vi "GeoData.vi"() -> ()   [LabVIEW 2017] (continued)
\tPembine\tWI\tMarinette County\tH1\n54151\t55075\tNiagara\tWI\tMarinette County\tH1\n54153\t55075\tOconto\tWI\tMarinette County\tH1\n54112\t55075\tColeman\tWI\tMarinette County\tH1\n54125\t55075\tGoodman\tWI\tMarinette County\tH1\n54119\t55075\tDunbar\tWI\tMarinette County\tH1\n54143\t55075\tMarinette\tWI\tMarinette County\tH1\n54139\t55075\tLena\tWI\tMarinette County\tH1\n54120\t55075\tFence\tWI\tMarinette County\tH1\n54159\t55075\tPorterfield\tWI\tMarinette County\tH1\n54103\t55075\tArmstrong creek\tWI\tMarinette County\tH1\n54114\t55075\tCrivitz\tWI\tMarinette County\tH1\n54102\t55075\tAmberg\tWI\tMarinette County\tH1\n54177\t55075\tWausaukee\tWI\tMarinette County\tH1\n54104\t55075\tAthelstane\tWI\tMarinette County\tH1\n53949\t55077\tMontello\tWI\tMarquette County\tH1\n53953\t55077\tPackwaukee\tWI\tMarquette County\tH1\n53954\t55077\tPardeeville\tWI\tMarquette County\tH1\n53930\t55077\tEndeavor\tWI\tMarquette County\tH1\n54930\t55077\tColoma\tWI\tMarquette County\tH1\n53946\t55077\tMarkesan\tWI\tMarquette County\tH1\n53920\t55077\tBriggsville\tWI\tMarquette County\tH1\n53901\t55077\tPortage\tWI\tMarquette County\tH1\n53952\t55077\tOxford\tWI\tMarquette County\tH1\n53926\t55077\tDalton\tWI\tMarquette County\tH1\n54960\t55077\tNeshkoro\tWI\tMarquette County\tH1\n54982\t55077\tWautoma\tWI\tMarquette County\tH1\n54968\t55077\tPrinceton\tWI\tMarquette County\tH1\n53964\t55077\tWestfield\tWI\tMarquette County\tH1\n54135\t55078\tKeshena\tWI\tMenominee County\tH1\n54166\t55078\tShawano\tWI\tMenominee County\tH1\n54174\t55078\tSuring\tWI\tMenominee County\tH1\n54124\t55078\tGillett\tWI\tMenominee County\tH1\n54150\t55078\tNeopit\tWI\tMenominee County\tH1\n53217\t55079\tMilwaukee\tWI\tMilwaukee County\tH1\n53220\t55079\tMilwaukee\tWI\tMilwaukee County\tH1\n53235\t55079\tSaint francis\tWI\tMilwaukee County\tH1\n53226\t55079\tMilwaukee\tWI\tMilwaukee County\tH1\n53221\t55079\tMilwaukee\tWI\tMilwaukee County\tH1\n53154\t55079\tOak creek\tWI\tMilwaukee County\tH1\n53204\t55079\tMilwaukee\tWI\tMilwaukee County\tH1\n53132\t55079\tFranklin\tWI\tMilwaukee County\tH1\n53219\t55079\tMilwaukee\tWI\tMilwaukee County\tH1\n53203\t55079\tMilwaukee\tWI\tMilwaukee County\tH1\n53207\t55079\tMilwaukee\tWI\tMilwaukee County\tH1\n53212\t55079\tMilwaukee\tWI\tMilwaukee County\tH1\n53007\t55079\tButler\tWI\tMilwaukee County\tH1\n53233\t55079\tMilwaukee\tWI\tMilwaukee County\tH1\n53202\t55079\tMilwaukee\tWI\tMilwaukee County\tH1\n53206\t55079\tMilwaukee\tWI\tMilwaukee County\tH1\n53172\t55079\tSouth milwaukee\tWI\tMilwaukee County\tH1\n53210\t55079\tMilwaukee\tWI\tMilwaukee County\tH1\n53215\t55079\tMilwaukee\tWI\tMilwaukee County\tH1\n53263\t55079\tMilwaukee\tWI\tMilwaukee County\tH1\n53129\t55079\tGreendale\tWI\tMilwaukee County\tH1\n53228\t55079\tMilwaukee\tWI\tMilwaukee County\tH1\n53216\t55079\tMilwaukee\tWI\tMilwaukee County\tH1\n53234\t55079\tMilwaukee\tWI\tMilwaukee County\tH1\n53237\t55079\tMilwaukee\tWI\tMilwaukee County\tH1\n53213\t55079\tMilwaukee\tWI\tMilwaukee County\tH1\n53201\t55079\tMilwaukee\tWI\tMilwaukee County\tH1\n53293\t55079\tMilwaukee\tWI\tMilwaukee County\tH1\n53274\t55079\tMilwaukee\tWI\tMilwaukee County\tH1\n53110\t55079\tCudahy\tWI\tMilwaukee County\tH1\n53130\t55079\tHales corners\tWI\tMilwaukee County\tH1\n53126\t55079\tFranksville\tWI\tMilwaukee County\tH1\n53225\t55079\tMilwaukee\tWI\tMilwaukee County\tH1\n53224\t55079\tMilwaukee\tWI\tMilwaukee County\tH1\n53223\t55079\tMilwaukee\tWI\tMilwaukee County\tH1\n53211\t55079\tMilwaukee\tWI\tMilwaukee County\tH1\n53214\t55079\tMilwaukee\tWI\tMilwaukee County\tH1\n53295\t55079\tMilwaukee\tWI\tMilwaukee County\tH1\n53278\t55079\tMilwaukee\tWI\tMilwaukee County\tH1\n53222\t55079\tMilwaukee\tWI\tMilwaukee County\tH1\n53209\t55079\tMilwaukee\tWI\tMilwaukee County\tH1\n53208\t55079\tMilwaukee\tWI\tMilwaukee County\tH1\n53218\t55079\tMilwaukee\tWI\tMilwaukee County\tH1\n53227\t55079\tMilwaukee\tWI\tMilwaukee County\tH1\n53205\t55079\tMilwaukee\tWI\tMilwaukee County\tH1\n53259\t55079\tMilwaukee\tWI\tMilwaukee County\tH1\n54618\t55081\tCamp douglas\tWI\tMonroe County\tH1\n54666\t55081\tWarrens\tWI\tMonroe County\tH1\n54648\t55081\tNorwalk\tWI\tMonroe County\tH1\n54651\t55081\tOntario\tWI\tMonroe County\tH1\n53929\t55081\tElroy\tWI\tMonroe County\tH1\n54670\t55081\tWilton\tWI\tMonroe County\tH1\n54660\t55081\tTomah\tWI\tMonroe County\tH1\n54656\t55081\tSparta\tWI\tMonroe County\tH1\n54653\t55081\tRockland\tWI\tMonroe County\tH1\n54649\t55081\tOakdale\tWI\tMonroe County\tH1\n54619\t55081\tCashton\tWI\tMonroe County\tH1\n54615\t55081\tBlack river falls\tWI\tMonroe County\tH1\n54662\t55081\tTunnel city\tWI\tMonroe County\tH1\n54614\t55081\tBangor\tWI\tMonroe County\tH1\n54638\t55081\tKendall\tWI\tMonroe County\tH1\n54620\t55081\tCataract\tWI\tMonroe County\tH1\n54157\t55083\tPeshtigo\tWI\tOconto County\tH1\n54111\t55083\tCecil\tWI\tOconto County\tH1\n54161\t55083\tPound\tWI\tOconto County\tH1\n54491\t55083\tWhite lake\tWI\tOconto County\tH1\n54153\t55083\tOconto\tWI\tOconto County\tH1\n54112\t55083\tColeman\tWI\tOconto County\tH1\n54137\t55083\tKrakow\tWI\tOconto County\tH1\n54174\t55083\tSuring\tWI\tOconto County\tH1\n54171\t55083\tSobieski\tWI\tOconto County\tH1\n54141\t55083\tLittle suamico\tWI\tOconto County\tH1\n54124\t55083\tGillett\tWI\tOconto County\tH1\n54149\t55083\tMountain\tWI\tOconto County\tH1\n54154\t55083\tOconto falls\tWI\tOconto County\tH1\n54139\t55083\tLena\tWI\tOconto County\tH1\n54175\t55083\tTownsend\tWI\tOconto County\tH1\n54101\t55083\tAbrams\tWI\tOconto County\tH1\n54114\t55083\tCrivitz\tWI\tOconto County\tH1\n54162\t55083\tPulaski\tWI\tOconto County\tH1\n54138\t55083\tLakewood\tWI\tOconto County\tH1\n54104\t55083\tAthelstane\tWI\tOconto County\tH1\n54538\t55085\tLac du flambeau\tWI\tOneida County\tH1\n54529\t55085\tHarshaw\tWI\tOneida County\tH1\n54564\t55085\tTripoli\tWI\tOneida County\tH1\n54543\t55085\tMc naughton\tWI\tOneida County\tH1\n54539\t55085\tLake tomahawk\tWI\tOneida County\tH1\n54558\t55085\tSaint germain\tWI\tOneida County\tH1\n54521\t55085\tEagle river\tWI\tOneida County\tH1\n54501\t55085\tRhinelander\tWI\tOneida County\tH1\n54428\t55085\tElcho\tWI\tOneida County\tH1\n54562\t55085\tThree lakes\tWI\tOneida County\tH1\n54548\t55085\tMinocqua\tWI\tOneida County\tH1\n54531\t55085\tHazelhurst\tWI\tOneida County\tH1\n54463\t55085\tPelican lake\tWI\tOneida County\tH1\n54568\t55085\tWoodruff\tWI\tOneida County\tH1\n54435\t55085\tGleason\tWI\tOneida County\tH1\n54487\t55085\tTomahawk\tWI\tOneida County\tH1\n54520\t55085\tCrandon\tWI\tOneida County\tH1\n54914\t55087\tAppleton\tWI\tOutagamie County\tH1\n54942\t55087\tGreenville\tWI\tOutagamie County\tH1\n54130\t55087\tKaukauna\tWI\tOutagamie County\tH1\n54155\t55087\tOneida\tWI\tOutagamie County\tH1\n54152\t55087\tNichols\tWI\tOutagamie County\tH1\n54180\t55087\tWrightstown\tWI\tOutagamie County\tH1\n54922\t55087\tBear creek\tWI\tOutagamie County\tH1\n54961\t55087\tNew london\tWI\tOutagamie County\tH1\n54940\t55087\tFremont\tWI\tOutagamie County\tH1\n54106\t55087\tBlack creek\tWI\tOutagamie County\tH1\n54956\t55087\tNeenah\tWI\tOutagamie County\tH1\n54115\t55087\tDe pere\tWI\tOutagamie County\tH1\n54913\t55087\tAppleton\tWI\tOutagamie County\tH1\n54107\t55087\tBonduel\tWI\tOutagamie County\tH1\n54113\t55087\tCombined locks\tWI\tOutagamie County\tH1\n54313\t55087\tGreen bay\tWI\tOutagamie County\tH1\n54919\t55087\tAppleton\tWI\tOutagamie County\tH1\n54136\t55087\tKimberly\tWI\tOutagamie County\tH1\n54140\t55087\tLittle chute\tWI\tOutagamie County\tH1\n54165\t55087\tSeymour\tWI\tOutagamie County\tH1\n54911\t55087\tAppleton\tWI\tOutagamie County\tH1\n54915\t55087\tAppleton\tWI\tOutagamie County\tH1\n54931\t55087\tDale\tWI\tOutagamie County\tH1\n54170\t55087\tShiocton\tWI\tOutagamie County\tH1\n54929\t55087\tClintonville\tWI\tOutagamie County\tH1\n54944\t55087\tHortonville\tWI\tOutagamie County\tH1\n54912\t55087\tAppleton\tWI\tOutagamie County\tH1\n53080\t55089\tSaukville\tWI\tOzaukee County\tH1\n53217\t55089\tMilwaukee\tWI\tOzaukee County\tH1\n53021\t55089\tFredonia\tWI\tOzaukee County\tH1\n53097\t55089\tMequon\tWI\tOzaukee County\tH1\n53024\t55089\tGrafton\tWI\tOzaukee County\tH1\n53092\t55089\tMequon\tWI\tOzaukee County\tH1\n53075\t55089\tRandom lake\tWI\tOzaukee County\tH1\n53004\t55089\tBelgium\tWI\tOzaukee County\tH1\n53012\t55089\tCedarburg\tWI\tOzaukee County\tH1\n53022\t55089\tGermantown\tWI\tOzaukee County\tH1\n53090\t55089\tWest bend\tWI\tOzaukee County\tH1\n53013\t55089\tCedar grove\tWI\tOzaukee County\tH1\n53095\t55089\tWest bend\tWI\tOzaukee County\tH1\n53074\t55089\tPort washington\tWI\tOzaukee County\tH1\n54721\t55091\tArkansaw\tWI\tPepin County\tH1\n54761\t55091\tPlum city\tWI\tPepin County\tH1\n54736\t55091\tDurand\tWI\tPepin County\tH1\n54737\t55091\tEau galle\tWI\tPepin County\tH1\n54755\t55091\tMondovi\tWI\tPepin County\tH1\n54759\t55091\tPepin\tWI\tPepin County\tH1\n54769\t55091\tStockholm\tWI\tPepin County\tH1\n54721\t55093\tArkansaw\tWI\tPierce County\tH1\n54011\t55093\tEllsworth\tWI\tPierce County\tH1\n54021\t55093\tPrescott\tWI\tPierce County\tH1\n54750\t55093\tMaiden rock\tWI\tPierce County\tH1\n54723\t55093\tBay city\tWI\tPierce County\tH1\n54761\t55093\tPlum city\tWI\tPierce County\tH1\n54005\t55093\tClear lake\tWI\tPierce County\tH1\n54014\t55093\tHager city\tWI\tPierce County\tH1\n54740\t55093\tElmwood\tWI\tPierce County\tH1\n54002\t55093\tBaldwin\tWI\tPierce County\tH1\n54003\t55093\tBeldenville\tWI\tPierce County\tH1\n54767\t55093\tSpring valley\tWI\tPierce County\tH1\n54022\t55093\tRiver falls\tWI\tPierce County\tH1\n54759\t55093\tPepin\tWI\tPierce County\tH1\n54769\t55093\tStockholm\tWI\tPierce County\tH1\n54004\t55095\tClayton\tWI\tPolk County\tH1\n54009\t55095\tDresser\tWI\tPolk County\tH1\n54858\t55095\tMilltown\tWI\tPolk County\tH1\n54826\t55095\tComstock\tWI\tPolk County\tH1\n54889\t55095\tTurtle lake\tWI\tPolk County\tH1\n54837\t55095\tFrederic\tWI\tPolk County\tH1\n54007\t55095\tDeer park\tWI\tPolk County\tH1\n54840\t55095\tGrantsburg\tWI\tPolk County\tH1\n54025\t55095\tSomerset\tWI\tPolk County\tH1\n54024\t55095\tSaint croix falls\tWI\tPolk County\tH1\n54006\t55095\tCushing\tWI\tPolk County\tH1\n54005\t55095\tClear lake\tWI\tPolk County\tH1\n54872\t55095\tSiren\tWI\tPolk County\tH1\n54026\t55095\tStar prairie\tWI\tPolk County\tH1\n54017\t55095\tNew richmond\tWI\tPolk County\tH1\n54001\t55095\tAmery\tWI\tPolk County\tH1\n54020\t55095\tOsceola\tWI\tPolk County\tH1\n54810\t55095\tBalsam lake\tWI\tPolk County\tH1\n54829\t55095\tCumberland\tWI\tPolk County\tH1\n54853\t55095\tLuck\tWI\tPolk County\tH1\n54824\t55095\tCenturia\tWI\tPolk County\tH1\n54482\t55097\tStevens point\tWI\tPortage County\tH1\n54407\t55097\tAmherst junction\tWI\tPortage County\tH1\n54455\t55097\tMosinee\tWI\tPortage County\tH1\n54473\t55097\tRosholt\tWI\tPortage County\tH1\n54423\t55097\tCuster\tWI\tPortage County\tH1\n54492\t55097\tStevens point\tWI\tPortage County\tH1\n54475\t55097\tRudolph\tWI\tPortage County\tH1\n54966\t55097\tPlainfield\tWI\tPortage County\tH1\n54443\t55097\tJunction city\tWI\tPortage County\tH1\n54945\t55097\tIola\tWI\tPortage County\tH1\n54984\t55097\tWild rose\tWI\tPortage County\tH1\n54481\t55097\tStevens point\tWI\tPortage County\tH1\n54921\t55097\tBancroft\tWI\tPortage County\tH1\n54458\t55097\tNelsonville\tWI\tPortage County\tH1\n54406\t55097\tAmherst\tWI\tPortage County\tH1\n54454\t55097\tMilladore\tWI\tPortage County\tH1\n54494\t55097\tWisconsin rapids\tWI\tPortage County\tH1\n54467\t55097\tPlover\tWI\tPortage County\tH1\n54909\t55097\tAlmond\tWI\tPortage County\tH1\n54981\t55097\tWaupaca\tWI\tPortage County\tH1\n54499\t55097\tWittenberg\tWI\tPortage County\tH1\n54977\t55097\tScandinavia\tWI\tPortage County\tH1\n54538\t55099\tLac du flambeau\tWI\tPrice County\tH1\n54490\t55099\tWestboro\tWI\tPrice County\tH1\n54513\t55099\tBrantwood\tWI\tPrice County\tH1\n54515\t55099\tCatawba\tWI\tPrice County\tH1\n54564\t55099\tTripoli\tWI\tPrice County\tH1\n54537\t55099\tKennan\tWI\tPrice County\tH1\n54459\t55099\tOgema\tWI\tPrice County\tH1\n54470\t55099\tRib lake\tWI\tPrice County\tH1\n54555\t55099\tPhillips\tWI\tPrice County\tH1\n54530\t55099\tHawkins\tWI\tPrice County\tH1\n54514\t55099\tButternut\tWI\tPrice County\tH1\n54552\t55099\tPark falls\tWI\tPrice County\tH1\n54524\t55099\tFifield\tWI\tPrice County\tH1\n54556\t55099\tPrentice\tWI\tPrice County\tH1\n53404\t55101\tRacine\tWI\tRacine County\tH1\n53144\t55101\tKenosha\tWI\tRacine County\tH1\n53105\t55101\tBurlington\tWI\tRacine County\tH1\n53402\t55101\tRacine\tWI\tRacine County\tH1\n53403\t55101\tRacine\tWI\tRacine County\tH1\n53408\t55101\tRacine\tWI\tRacine County\tH1\n53182\t55101\tUnion grove\tWI\tRacine County\tH1\n53185\t55101\tWaterford\tWI\tRacine County\tH1\n53149\t55101\tMukwonago\tWI\tRacine County\tH1\n53138\t55101\tHoney creek\tWI\tRacine County\tH1\n53401\t55101\tRacine\tWI\tRacine County\tH1\n53167\t55101\tRochester\tWI\tRacine County\tH1\n53120\t55101\tEast troy\tWI\tRacine County\tH1\n53108\t55101\tCaledonia\tWI\tRacine County\tH1\n53126\t55101\tFranksville\tWI\tRacine County\tH1\n53150\t55101\tMuskego\tWI\tRacine County\tH1\n53177\t55101\tSturtevant\tWI\tRacine County\tH1\n53405\t55101\tRacine\tWI\tRacine County\tH1\n53406\t55101\tRacine\tWI\tRacine County\tH1\n53139\t55101\tKansasville\tWI\tRacine County\tH1\n53556\t55103\tLone rock\tWI\tRichland County\tH1\n53968\t55103\tWonewoc\tWI\tRichland County\tH1\n53937\t55103\tHillpoint\tWI\tRichland County\tH1\n54634\t55103\tHillsboro\tWI\tRichland County\tH1\n54664\t55103\tViola\tWI\tRichland County\tH1\n53573\t55103\tMuscoda\tWI\tRichland County\tH1\n54655\t55103\tSoldiers grove\tWI\tRichland County\tH1\n53584\t55103\tSextonville\tWI\tRichland County\tH1\n53540\t55103\tGotham\tWI\tRichland County\tH1\n53518\t55103\tBlue river\tWI\tRichland County\tH1\n54639\t55103\tLa farge\tWI\tRichland County\tH1\n53581\t55103\tRichland center\tWI\tRichland County\tH1\n53588\t55103\tSpring green\tWI\tRichland County\tH1\n53805\t55103\tBoscobel\tWI\tRichland County\tH1\n53924\t55103\tCazenovia\tWI\tRichland County\tH1\n53941\t55103\tLa valle\tWI\tRichland County\tH1\n53545\t55105\tJanesville\tWI\tRock County\tH1\n53521\t55105\tBrooklyn\tWI\tRock County\tH1\n53502\t55105\tAlbany\tWI\tRock County\tH1\n53537\t55105\tFootville\tWI\tRock County\tH1\n53563\t55105\tMilton\tWI\tRock County\tH1\n53525\t55105\tClinton\tWI\tRock County\tH1\n53520\t55105\tBrodhead\tWI\tRock County\tH1\n53536\t55105\tEvansville\tWI\tRock County\tH1\n53190\t55105\tWhitewater\tWI\tRock County\tH1\n53501\t55105\tAfton\tWI\tRock County\tH1\n53511\t55105\tBeloit\tWI\tRock County\tH1\n53576\t55105\tOrfordville\tWI\tRock County\tH1\n53547\t55105\tJanesville\tWI\tRock County\tH1\n53505\t55105\tAvalon\tWI\tRock County\tH1\n53114\t55105\tDarien\tWI\tRock County\tH1\n53585\t55105\tSharon\tWI\tRock County\tH1\n53589\t55105\tStoughton\tWI\tRock County\tH1\n53512\t55105\tBeloit\tWI\tRock County\tH1\n53538\t55105\tFort atkinson\tWI\tRock County\tH1\n53546\t55105\tJanesville\tWI\tRock County\tH1\n53548\t55105\tJanesville\tWI\tRock County\tH1\n53534\t55105\tEdgerton\tWI\tRock County\tH1\n54526\t55107\tGlen flora\tWI\tRusk County\tH1\n54835\t55107\tExeland\tWI\tRusk County\tH1\n54728\t55107\tChetek\tWI\tRusk County\tH1\n54745\t55107\tHolcombe\tWI\tRusk County\tH1\n54757\t55107\tNew auburn\tWI\tRusk County\tH1\n54563\t55107\tTony\tWI\tRusk County\tH1\n54848\t55107\tLadysmith\tWI\tRusk County\tH1\n54868\t55107\tRice lake\tWI\tRusk County\tH1\n54895\t55107\tWeyerhaeuser\tWI\tRusk County\tH1\n54530\t55107\tHawkins\tWI\tRusk County\tH1\n54819\t55107\tBruce\tWI\tRusk County\tH1\n54731\t55107\tConrath\tWI\tRusk County\tH1\n54766\t55107\tSheldon\tWI\tRusk County\tH1\n54817\t55107\tBirchwood\tWI\tRusk County\tH1\n54028\t55109\tWoodville\tWI\tSt. Croix County\tH1\n54749\t55109\tKnapp\tWI\tSt. Croix County\tH1\n54027\t55109\tWilson\tWI\tSt. Croix County\tH1\n54751\t55109\tMenomonie\tWI\tSt. Croix County\tH1\n54023\t55109\tRoberts\tWI\tSt. Croix County\tH1\n54007\t55109\tDeer park\tWI\tSt. Croix County\tH1\n54015\t55109\tHammond\tWI\tSt. Croix County\tH1\n54082\t55109\tHoulton\tWI\tSt. Croix County\tH1\n54013\t55109\tGlenwood city\tWI\tSt. Croix County\tH1\n54025\t55109\tSomerset\tWI\tSt. Croix County\tH1\n54005\t55109\tClear lake\tWI\tSt. Croix County\tH1\n54026\t55109\tStar prairie\tWI\tSt. Croix County\tH1\n54002\t55109\tBaldwin\tWI\tSt. Croix County\tH1\n54016\t55109\tHudson\tWI\tSt. Croix County\tH1\n54017\t55109\tNew richmond\tWI\tSt. Croix County\tH1\n54734\t55109\tDowning\tWI\tSt. Croix County\tH1\n54767\t55109\tSpring valley\tWI\tSt. Croix County\tH1\n54022\t55109\tRiver falls\tWI\tSt. Croix County\tH1\n54020\t55109\tOsceola\tWI\tSt. Croix County\tH1\n53556\t55111\tLone rock\tWI\tSauk County\tH1\n53968\t55111\tWonewoc\tWI\tSauk County\tH1\n53937\t55111\tHillpoint\tWI\tSauk County\tH1\n53959\t55111\tReedsburg\tWI\tSauk County\tH1\n53561\t55111\tMerrimac\tWI\tSauk County\tH1\n53961\t55111\tRock springs\tWI\tSauk County\tH1\n53942\t55111\tLime ridge\tWI\tSauk County\tH1\n53901\t55111\tPortage\tWI\tSauk County\tH1\n53944\t55111\tLyndon station\tWI\tSauk County\tH1\n53958\t55111\tReedsburg\tWI\tSauk County\tH1\n53577\t55111\tPlain\tWI\tSauk County\tH1\n53965\t55111\tWisconsin dells\tWI\tSauk County\tH1\n53943\t55111\tLoganville\tWI\tSauk County\tH1\n53583\t55111\tSauk city\tWI\tSauk County\tH1\n53588\t55111\tSpring green\tWI\tSauk County\tH1\n53578\t55111\tPrairie du sac\tWI\tSauk County\tH1\n53913\t55111\tBaraboo\tWI\tSauk County\tH1\n53951\t55111\tNorth freedom\tWI\tSauk County\tH1\n53924\t55111\tCazenovia\tWI\tSauk County\tH1\n53941\t55111\tLa valle\tWI\tSauk County\tH1\n53940\t55111\tLake delton\tWI\tSauk County\tH1\n54876\t55113\tStone lake\tWI\tSawyer County\tH1\n54835\t55113\tExeland\tWI\tSawyer County\tH1\n54843\t55113\tHayward\tWI\tSawyer County\tH1\n54821\t55113\tCable\tWI\tSawyer County\tH1\n54867\t55113\tRadisson\tWI\tSawyer County\tH1\n54555\t55113\tPhillips\tWI\tSawyer County\tH1\n54862\t55113\tOjibwa\tWI\tSawyer County\tH1\n54828\t55113\tCouderay\tWI\tSawyer County\tH1\n54552\t55113\tPark falls\tWI\tSawyer County\tH1\n54896\t55113\tWinter\tWI\tSawyer County\tH1\n54817\t55113\tBirchwood\tWI\tSawyer County\tH1\n54166\t55115\tShawano\tWI\tShawano County\tH1\n54111\t55115\tCecil\tWI\tShawano County\tH1\n54486\t55115\tTigerton\tWI\tShawano County\tH1\n54450\t55115\tMattoon\tWI\tShawano County\tH1\n54106\t55115\tBlack creek\tWI\tShawano County\tH1\n54137\t55115\tKrakow\tWI\tShawano County\tH1\n54408\t55115\tAniwa\tWI\tShawano County\tH1\n54928\t55115\tCaroline\tWI\tShawano County\tH1\n54978\t55115\tTilleda\tWI\tShawano County\tH1\n54124\t55115\tGillett\tWI\tShawano County\tH1\n54154\t55115\tOconto falls\tWI\tShawano County\tH1\n54107\t55115\tBonduel\tWI\tShawano County\tH1\n54427\t55115\tEland\tWI\tShawano County\tH1\n54127\t55115\tGreen valley\tWI\tShawano County\tH1\n54128\t55115\tGresham\tWI\tShawano County\tH1\n54409\t55115\tAntigo\tWI\tShawano County\tH1\n54948\t55115\tLeopolis\tWI\tShawano County\tH1\n54165\t55115\tSeymour\tWI\tShawano County\tH1\n54950\t55115\tMarion\tWI\tShawano County\tH1\n54162\t55115\tPulaski\tWI\tShawano County\tH1\n54170\t55115\tShiocton\tWI\tShawano County\tH1\n54416\t55115\tBowler\tWI\tShawano County\tH1\n54414\t55115\tBirnamwood\tWI\tShawano County\tH1\n54499\t55115\tWittenberg\tWI\tShawano County\tH1\n54929\t55115\tClintonville\tWI\tShawano County\tH1\n53085\t55117\tSheboygan falls\tWI\tSheboygan County\tH1\n53044\t55117\tKohler\tWI\tSheboygan County\tH1\n53073\t55117\tPlymouth\tWI\tSheboygan County\tH1\n53081\t55117\tSheboygan\tWI\tSheboygan County\tH1\n53083\t55117\tSheboygan\tWI\tSheboygan County\tH1\n53021\t55117\tFredonia\tWI\tSheboygan County\tH1\n53093\t55117\tWaldo\tWI\tSheboygan County\tH1\n53015\t55117\tCleveland\tWI\tSheboygan County\tH1\n53042\t55117\tKiel\tWI\tSheboygan County\tH1\n53023\t55117\tGlenbeulah\tWI\tSheboygan County\tH1\n53082\t55117\tSheboygan\tWI\tSheboygan County\tH1\n53075\t55117\tRandom lake\tWI\tSheboygan County\tH1\n53070\t55117\tOostburg\tWI\tSheboygan County\tH1\n53079\t55117\tSaint cloud\tWI\tSheboygan County\tH1\n53001\t55117\tAdell\tWI\tSheboygan County\tH1\n53004\t55117\tBelgium\tWI\tSheboygan County\tH1\n53026\t55117\tGreenbush\tWI\tSheboygan County\tH1\n53011\t55117\tCascade\tWI\tSheboygan County\tH1\n53031\t55117\tHingham\tWI\tSheboygan County\tH1\n53020\t55117\tElkhart lake\tWI\tSheboygan County\tH1\n53013\t55117\tCedar grove\tWI\tSheboygan County\tH1\n53040\t55117\tKewaskum\tWI\tSheboygan County\tH1\n54771\t55119\tThorp\tWI\tTaylor County\tH1\n54451\t55119\tMedford\tWI\tTaylor County\tH1\n54425\t55119\tDorchester\tWI\tTaylor County\tH1\n54490\t55119\tWestboro\tWI\tTaylor County\tH1\n54498\t55119\tWithee\tWI\tTaylor County\tH1\n54459\t55119\tOgema\tWI\tTaylor County\tH1\n54460\t55119\tOwen\tWI\tTaylor County\tH1\n54470\t55119\tRib lake\tWI\tTaylor County\tH1\n54411\t55119\tAthens\tWI\tTaylor County\tH1\n54447\t55119\tLublin\tWI\tTaylor County\tH1\n54433\t55119\tGilman\tWI\tTaylor County\tH1\n54480\t55119\tStetsonville\tWI\tTaylor County\tH1\n54768\t55119\tStanley\tWI\tTaylor County\tH1\n54766\t55119\tSheldon\tWI\tTaylor County\tH1\n54422\t55119\tCurtiss\tWI\tTaylor County\tH1\n54770\t55121\tStrum\tWI\tTrempealeau County\tH1\n54661\t55121\tTrempealeau\tWI\tTrempealeau County\tH1\n54612\t55121\tArcadia\tWI\tTrempealeau County\tH1\n54642\t55121\tMelrose\tWI\tTrempealeau County\tH1\n54738\t55121\tEleva\tWI\tTrempealeau County\tH1\n54747\t55121\tIndependence\tWI\tTrempealeau County\tH1\n54625\t55121\tDodge\tWI\tTrempealeau County\tH1\n54659\t55121\tTaylor\tWI\tTrempealeau County\tH1\n54630\t55121\tGalesville\tWI\tTrempealeau County\tH1\n54616\t55121\tBlair\tWI\tTrempealeau County\tH1\n54758\t55121\tOsseo\tWI\tTrempealeau County\tH1\n54773\t55121\tWhitehall\tWI\tTrempealeau County\tH1\n54760\t55121\tPigeon falls\tWI\tTrempealeau County\tH1\n54627\t55121\tEttrick\tWI\tTrempealeau County\tH1\n54755\t55121\tMondovi\tWI\tTrempealeau County\tH1\n53968\t55123\tWonewoc\tWI\tVernon County\tH1\n54634\t55123\tHillsboro\tWI\tVernon County\tH1\n54667\t55123\tWestby\tWI\tVernon County\tH1\n54664\t55123\tViola\tWI\tVernon County\tH1\n54651\t55123\tOntario\tWI\tVernon County\tH1\n53929\t55123\tElroy\tWI\tVernon County\tH1\n54621\t55123\tChaseburg\tWI\tVernon County\tH1\n54623\t55123\tCoon valley\tWI\tVernon County\tH1\n54658\t55123\tStoddard\tWI\tVernon County\tH1\n54655\t55123\tSoldiers grove\tWI\tVernon County\tH1\n54619\t55123\tCashton\tWI\tVernon County\tH1\n54639\t55123\tLa farge\tWI\tVernon County\tH1\n54624\t55123\tDe soto\tWI\tVernon County\tH1\n54665\t55123\tViroqua\tWI\tVernon County\tH1\n54632\t55123\tGenoa\tWI\tVernon County\tH1\n54638\t55123\tKendall\tWI\tVernon County\tH1\n54652\t55123\tReadstown\tWI\tVernon County\tH1\n54628\t55123\tFerryville\tWI\tVernon County\tH1\n54538\t55125\tLac du flambeau\tWI\tVilas County\tH1\n54554\t55125\tPhelps\tWI\tVilas County\tH1\n54560\t55125\tSayner\tWI\tVilas County\tH1\n54558\t55125\tSaint germain\tWI\tVilas County\tH1\n54521\t55125\tEagle river\tWI\tVilas County\tH1\n54519\t55125\tConover\tWI\tVilas County\tH1\n54540\t55125\tLand o lakes\tWI\tVilas County\tH1\n54548\t55125\tMinocqua\tWI\tVilas County\tH1\n54545\t55125\tManitowish waters\tWI\tVilas County\tH1\n54512\t55125\tBoulder junction\tWI\tVilas County\tH1\n54568\t55125\tWoodruff\tWI\tVilas County\tH1\n54561\t55125\tStar lake\tWI\tVilas County\tH1\n54557\t55125\tPresque isle\tWI\tVilas County\tH1\n53125\t55127\tFontana\tWI\tWalworth County\tH1\n53128\t55127\tGenoa city\tWI\tWalworth County\tH1\n53184\t55127\tWalworth\tWI\tWalworth County\tH1\n53105\t55127\tBurlington\tWI\tWalworth County\tH1\n53525\t55127\tClinton\tWI\tWalworth County\tH1\n53149\t55127\tMukwonago\tWI\tWalworth County\tH1\n53190\t55127\tWhitewater\tWI\tWalworth County\tH1\n53176\t55127\tSpringfield\tWI\tWalworth County\tH1\n53120\t55127\tEast troy\tWI\tWalworth County\tH1\n53114\t55127\tDarien\tWI\tWalworth County\tH1\n53585\t55127\tSharon\tWI\tWalworth County\tH1\n53147\t55127\tLake geneva\tWI\tWalworth County\tH1\n53156\t55127\tPalmyra\tWI\tWalworth County\tH1\n53119\t55127\tEagle\tWI\tWalworth County\tH1\n53191\t55127\tWilliams bay\tWI\tWalworth County\tH1\n53195\t55127\tZenda\tWI\tWalworth County\tH1\n53157\t55127\tPell lake\tWI\tWalworth County\tH1\n53115\t55127\tDelavan\tWI\tWalworth County\tH1\n53121\t55127\tElkhorn\tWI\tWalworth County\tH1\n53148\t55127\tLyons\tWI\tWalworth County\tH1\n54830\t55129\tDanbury\tWI\tWashburn County\tH1\n54813\t55129\tBarronett\tWI\tWashburn County\tH1\n54876\t55129\tStone lake\tWI\tWashburn County\tH1\n54843\t55129\tHayward\tWI\tWashburn County\tH1\n54868\t55129\tRice lake\tWI\tWashburn County\tH1\n54871\t55129\tShell lake\tWI\tWashburn County\tH1\n54888\t55129\tTrego\tWI\tWashburn County\tH1\n54801\t55129\tSpooner\tWI\tWashburn County\tH1\n54875\t55129\tSpringbrook\tWI\tWashburn County\tH1\n54870\t55129\tSarona\tWI\tWashburn County\tH1\n54859\t55129\tMinong\tWI\tWashburn County\tH1\n54817\t55129\tBirchwood\tWI\tWashburn County\tH1\n53080\t55131\tSaukville\tWI\tWashington County\tH1\n53027\t55131\tHartford\tWI\tWashington County\tH1\n53076\t55131\tRichfield\tWI\tWashington County\tH1\n53002\t55131\tAllenton\tWI\tWashington County\tH1\n53060\t55131\tNewburg\tWI\tWashington County\tH1\n53029\t55131\tHartland\tWI\tWashington County\tH1\n53066\t55131\tOconomowoc\tWI\tWashington County\tH1\n53033\t55131\tHubertus\tWI\tWashington County\tH1\n53010\t55131\tCampbellsport\tWI\tWashington County\tH1\n53021\t55131\tFredonia\tWI\tWashington County\tH1\n53091\t55131\tTheresa\tWI\tWashington County\tH1\n53017\t55131\tColgate\tWI\tWashington County\tH1\n53075\t55131\tRandom lake\tWI\tWashington County\tH1\n53086\t55131\tSlinger\tWI\tWashington County\tH1\n53012\t55131\tCedarburg\tWI\tWashington County\tH1\n53022\t55131\tGermantown\tWI\tWashington County\tH1\n53090\t55131\tWest bend\tWI\tWashington County\tH1\n53037\t55131\tJackson\tWI\tWashington County\tH1\n53095\t55131\tWest bend\tWI\tWashington County\tH1\n53040\t55131\tKewaskum\tWI\tWashington County\tH1\n53186\t55133\tWaukesha\tWI\tWaukesha County\tH1\n53018\t55133\tDelafield\tWI\tWaukesha County\tH1\n53069\t55133\tOkauchee\tWI\tWaukesha County\tH1\n53029\t55133\tHartland\tWI\tWaukesha County\tH1\n53066\t55133\tOconomowoc\tWI\tWaukesha County\tH1\n53072\t55133\tPewaukee\tWI\tWaukesha County\tH1\n53052\t55133\tMenomonee falls\tWI\tWaukesha County\tH1\n53122\t55133\tElm grove\tWI\tWaukesha County\tH1\n53185\t55133\tWaterford\tWI\tWaukesha County\tH1\n53149\t55133\tMukwonago\tWI\tWaukesha County\tH1\n53183\t55133\tWales\tWI\tWaukesha County\tH1\n53153\t55133\tNorth prairie\tWI\tWaukesha County\tH1\n53045\t55133\tBrookfield\tWI\tWaukesha County\tH1\n53132\t55133\tFranklin\tWI\tWaukesha County\tH1\n53007\t55133\tButler\tWI\tWaukesha County\tH1\n53008\t55133\tBrookfield\tWI\tWaukesha County\tH1\n53118\t55133\tDousman\tWI\tWaukesha County\tH1\n53017\t55133\tColgate\tWI\tWaukesha County\tH1\n53046\t55133\tLannon\tWI\tWaukesha County\tH1\n53058\t55133\tNashotah\tWI\tWaukesha County\tH1\n53036\t55133\tIxonia\tWI\tWaukesha County\tH1\n53127\t55133\tGenesee depot\tWI\tWaukesha County\tH1\n53228\t55133\tMilwaukee\tWI\tWaukesha County\tH1\n53151\t55133\tNew berlin\tWI\tWaukesha County\tH1\n53188\t55133\tWaukesha\tWI\tWaukesha County\tH1\n53056\t55133\tMerton\tWI\tWaukesha County\tH1\n53089\t55133\tSussex\tWI\tWaukesha County\tH1\n53225\t55133\tMilwaukee\tWI\tWaukesha County\tH1\n53150\t55133\tMuskego\tWI\tWaukesha County\tH1\n53005\t55133\tBrookfield\tWI\tWaukesha County\tH1\n53022\t55133\tGermantown\tWI\tWaukesha County\tH1\n53064\t55133\tNorth lake\tWI\tWaukesha County\tH1\n53103\t55133\tBig bend\tWI\tWaukesha County\tH1\n53119\t55133\tEagle\tWI\tWaukesha County\tH1\n53146\t55133\tNew berlin\tWI\tWaukesha County\tH1\n53051\t55133\tMenomonee falls\tWI\tWaukesha County\tH1\n53227\t55133\tMilwaukee\tWI\tWaukesha County\tH1\n53189\t55133\tWaukesha\tWI\tWaukesha County\tH1\n53187\t55133\tWaukesha\tWI\tWaukesha County\tH1\n54486\t55135\tTigerton\tWI\tWaupaca County\tH1\n54922\t55135\tBear creek\tWI\tWaupaca County\tH1\n54961\t55135\tNew london\tWI\tWaupaca County\tH1\n54962\t55135\tOgdensburg\tWI\tWaupaca County\tH1\n54940\t55135\tFremont\tWI\tWaupaca County\tH1\n54965\t55135\tPine river\tWI\tWaupaca County\tH1\n54933\t55135\tEmbarrass\tWI\tWaupaca County\tH1\n54742\t55135\tFall creek\tWI\tWaupaca County\tH1\n54945\t55135\tIola\tWI\tWaupaca County\tH1\n54983\t55135\tWeyauwega\tWI\tWaupaca County\tH1\n54990\t55135\tIola\tWI\tWaupaca County\tH1\n54981\t55135\tWaupaca\tWI\tWaupaca County\tH1\n54949\t55135\tManawa\tWI\tWaupaca County\tH1\n54950\t55135\tMarion\tWI\tWaupaca County\tH1\n54946\t55135\tKing\tWI\tWaupaca County\tH1\n54170\t55135\tShiocton\tWI\tWaupaca County\tH1\n54499\t55135\tWittenberg\tWI\tWaupaca County\tH1\n54929\t55135\tClintonville\tWI\tWaupaca County\tH1\n54977\t55135\tScandinavia\tWI\tWaupaca County\tH1\n54969\t55135\tReadfield\tWI\tWaupaca County\tH1\n54926\t55135\tBig falls\tWI\tWaupaca County\tH1\n54970\t55137\tRedgranite\tWI\tWaushara County\tH1\n54940\t55137\tFremont\tWI\tWaushara County\tH1\n54986\t55137\tWinneconne\tWI\tWaushara County\tH1\n54930\t55137\tColoma\tWI\tWaushara County\tH1\n54923\t55137\tBerlin\tWI\tWaushara County\tH1\n54965\t55137\tPine river\tWI\tWaushara County\tH1\n54966\t55137\tPlainfield\tWI\tWaushara County\tH1\n54943\t55137\tHancock\tWI\tWaushara County\tH1\n54984\t55137\tWild rose\tWI\tWaushara County\tH1\n54983\t55137\tWeyauwega\tWI\tWaushara County\tH1\n54976\t55137\tSaxeville\tWI\tWaushara County\tH1\n54921\t55137\tBancroft\tWI\tWaushara County\tH1\n54967\t55137\tPoy sippi\tWI\tWaushara County\tH1\n54909\t55137\tAlmond\tWI\tWaushara County\tH1\n54960\t55137\tNeshkoro\tWI\tWaushara County\tH1\n54982\t55137\tWautoma\tWI\tWaushara County\tH1\n54981\t55137\tWaupaca\tWI\tWaushara County\tH1\n53964\t55137\tWestfield\tWI\tWaushara County\tH1\n54963\t55137\tOmro\tWI\tWaushara County\tH1\n54904\t55139\tOshkosh\tWI\tWinnebago County\tH1\n54914\t55139\tAppleton\tWI\tWinnebago County\tH1\n54947\t55139\tLarsen\tWI\tWinnebago County\tH1\n54927\t55139\tButte des morts\tWI\tWinnebago County\tH1\n54940\t55139\tFremont\tWI\tWinnebago County\tH1\n54986\t55139\tWinneconne\tWI\tWinnebago County\tH1\n54956\t55139\tNeenah\tWI\tWinnebago County\tH1\n54979\t55139\tVan dyne\tWI\tWinnebago County\tH1\n54985\t55139\tWinnebago\tWI\tWinnebago County\tH1\n54901\t55139\tOshkosh\tWI\tWinnebago County\tH1\n54923\t55139\tBerlin\tWI\tWinnebago County\tH1\n54964\t55139\tPickett\tWI\tWinnebago County\tH1\n54971\t55139\tRipon\tWI\tWinnebago County\tH1\n54980\t55139\tWaukau\tWI\tWinnebago County\tH1\n54902\t55139\tOshkosh\tWI\tWinnebago County\tH1\n54903\t55139\tOshkosh\tWI\tWinnebago County\tH1\n54957\t55139\tNeenah\tWI\tWinnebago County\tH1\n54915\t55139\tAppleton\tWI\tWinnebago County\tH1\n54906\t55139\tOshkosh\tWI\tWinnebago County\tH1\n54952\t55139\tMenasha\tWI\tWinnebago County\tH1\n54963\t55139\tOmro\tWI\tWinnebago County\tH1\n54944\t55139\tHortonville\tWI\tWinnebago County\tH1\n54469\t55141\tPort edwards\tWI\tWood County\tH1\n54420\t55141\tChili\tWI\tWood County\tH1\n54412\t55141\tAuburndale\tWI\tWood County\tH1\n54495\t55141\tWisconsin rapids\tWI\tWood County\tH1\n54404\t55141\tMarshfield\tWI\tWood County\tH1\n54415\t55141\tBlenker\tWI\tWood County\tH1\n54475\t55141\tRudolph\tWI\tWood County\tH1\n54472\t55141\tMarshfield\tWI\tWood County\tH1\n54443\t55141\tJunction city\tWI\tWood County\tH1\n54441\t55141\tHewitt\tWI\tWood County\tH1\n54489\t55141\tVesper\tWI\tWood County\tH1\n54449\t55141\tMarshfield\tWI\tWood County\tH1\n54457\t55141\tNekoosa\tWI\tWood County\tH1\n54454\t55141\tMilladore\tWI\tWood County\tH1\n54410\t55141\tArpin\tWI\tWood County\tH1\n54494\t55141\tWisconsin rapids\tWI\tWood County\tH1\n54413\t55141\tBabcock\tWI\tWood County\tH1\n54466\t55141\tPittsville\tWI\tWood County\tH1\n82073\t56001\tLaramie\tWY\tAlbany County\tH1\n82058\t56001\tGarrett\tWY\tAlbany County\tH1\n82059\t56001\tGranite canon\tWY\tAlbany County\tH1\n82083\t56001\tRock river\tWY\tAlbany County\tH1\n82201\t56001\tWheatland\tWY\tAlbany County\tH1\n82052\t56001\tBuford\tWY\tAlbany County\tH1\n82071\t56001\tLaramie\tWY\tAlbany County\tH1\n82055\t56001\tCentennial\tWY\tAlbany County\tH1\n82063\t56001\tJelm\tWY\tAlbany County\tH1\n82084\t56001\tTie siding\tWY\tAlbany County\tH1\n82070\t56001\tLaramie\tWY\tAlbany County\tH1\n82072\t56001\tLaramie\tWY\tAlbany County\tH1\n82329\t56001\tMedicine bow\tWY\tAlbany County\tH1\n82051\t56001\tBosler\tWY\tAlbany County\tH1\n82423\t56003\tFrannie\tWY\tBig Horn County\tH1\n82421\t56003\tDeaver\tWY\tBig Horn County\tH1\n82428\t56003\tHyattville\tWY\tBig Horn County\tH1\n82422\t56003\tEmblem\tWY\tBig Horn County\tH1\n82442\t56003\tTen sleep\tWY\tBig Horn County\tH1\n82411\t56003\tBurlington\tWY\tBig Horn County\tH1\n82420\t56003\tCowley\tWY\tBig Horn County\tH1\n82412\t56003\tByron\tWY\tBig Horn County\tH1\n82401\t56003\tWorland\tWY\tBig Horn County\tH1\n82431\t56003\tLovell\tWY\tBig Horn County\tH1\n82410\t56003\tBasin\tWY\tBig Horn County\tH1\n82432\t56003\tManderson\tWY\tBig Horn County\tH1\n82426\t56003\tGreybull\tWY\tBig Horn County\tH1\n82441\t56003\tShell\tWY\tBig Horn County\tH1\n82435\t56003\tPowell\tWY\tBig Horn County\tH1\n82434\t56003\tOtto\tWY\tBig Horn County\tH1\n82701\t56005\tNewcastle\tWY\tCampbell County\tH1\n82727\t56005\tRozet\tWY\tCampbell County\tH1\n82732\t56005\tWright\tWY\tCampbell County\tH1\n82716\t56005\tGillette\tWY\tCampbell County\tH1\n82725\t56005\tRecluse\tWY\tCampbell County\tH1\n82731\t56005\tWeston\tWY\tCampbell County\tH1\n82831\t56005\tArvada\tWY\tCampbell County\tH1\n82721\t56005\tMoorcroft\tWY\tCampbell County\tH1\n82718\t56005\tGillette\tWY\tCampbell County\tH1\n82083\t56007\tRock river\tWY\tCarbon County\tH1\n82334\t56007\tSinclair\tWY\tCarbon County\tH1\n82615\t56007\tShirley basin\tWY\tCarbon County\tH1\n82324\t56007\tElk mountain\tWY\tCarbon County\tH1\n82325\t56007\tEncampment\tWY\tCarbon County\tH1\n82332\t56007\tSavery\tWY\tCarbon County\tH1\n82335\t56007\tWalcott\tWY\tCarbon County\tH1\n82301\t56007\tRawlins\tWY\tCarbon County\tH1\n82604\t56007\tCasper\tWY\tCarbon County\tH1\n82327\t56007\tHanna\tWY\tCarbon County\tH1\n82323\t56007\tDixon\tWY\tCarbon County\tH1\n82329\t56007\tMedicine bow\tWY\tCarbon County\tH1\n82331\t56007\tSaratoga\tWY\tCarbon County\tH1\n82321\t56007\tBaggs\tWY\tCarbon County\tH1\n82633\t56009\tDouglas\tWY\tConverse County\tH1\n82637\t56009\tGlenrock\tWY\tConverse County\tH1\n82224\t56009\tLost springs\tWY\tConverse County\tH1\n82636\t56009\tEvansville\tWY\tConverse County\tH1\n82229\t56009\tShawnee\tWY\tConverse County\tH1\n82729\t56011\tSundance\tWY\tCrook County\tH1\n82712\t56011\tBeulah\tWY\tCrook County\tH1\n82720\t56011\tHulett\tWY\tCrook County\tH1\n82721\t56011\tMoorcroft\tWY\tCrook County\tH1\n82714\t56011\tDevils tower\tWY\tCrook County\tH1\n82711\t56011\tAlva\tWY\tCrook County\tH1\n82730\t56011\tUpton\tWY\tCrook County\tH1\n82710\t56011\tAladdin\tWY\tCrook County\tH1\n82520\t56013\tLander\tWY\tFremont County\tH1\n82638\t56013\tHiland\tWY\tFremont County\tH1\n82513\t56013\tDubois\tWY\tFremont County\tH1\n82524\t56013\tSaint stephens\tWY\tFremont County\tH1\n82516\t56013\tKinnear\tWY\tFremont County\tH1\n82642\t56013\tLysite\tWY\tFremont County\tH1\n82310\t56013\tJeffrey city\tWY\tFremont County\tH1\n82649\t56013\tShoshoni\tWY\tFremont County\tH1\n82301\t56013\tRawlins\tWY\tFremont County\tH1\n82523\t56013\tPavillion\tWY\tFremont County\tH1\n82512\t56013\tCrowheart\tWY\tFremont County\tH1\n82514\t56013\tFort washakie\tWY\tFremont County\tH1\n82501\t56013\tRiverton\tWY\tFremont County\tH1\n82510\t56013\tArapahoe\tWY\tFremont County\tH1\n82515\t56013\tHudson\tWY\tFremont County\tH1\n82244\t56015\tYoder\tWY\tGoshen County\tH1\n82243\t56015\tVeteran\tWY\tGoshen County\tH1\n82221\t56015\tLagrange\tWY\tGoshen County\tH1\n82240\t56015\tTorrington\tWY\tGoshen County\tH1\n82201\t56015\tWheatland\tWY\tGoshen County\tH1\n82225\t56015\tLusk\tWY\tGoshen County\tH1\n82223\t56015\tLingle\tWY\tGoshen County\tH1\n82210\t56015\tChugwater\tWY\tGoshen County\tH1\n82242\t56015\tVan tassell\tWY\tGoshen County\tH1\n82217\t56015\tHawk springs\tWY\tGoshen County\tH1\n82219\t56015\tJay em\tWY\tGoshen County\tH1\n82212\t56015\tFort laramie\tWY\tGoshen County\tH1\n82218\t56015\tHuntley\tWY\tGoshen County\tH1\n82443\t56017\tThermopolis\tWY\tHot Springs County\tH1\n82430\t56017\tKirby\tWY\tHot Springs County\tH1\n82401\t56017\tWorland\tWY\tHot Springs County\tH1\n82832\t56019\tBanner\tWY\tJohnson County\tH1\n82835\t56019\tClearmont\tWY\tJohnson County\tH1\n82840\t56019\tSaddlestring\tWY\tJohnson County\tH1\n82834\t56019\tBuffalo\tWY\tJohnson County\tH1\n82831\t56019\tArvada\tWY\tJohnson County\tH1\n82640\t56019\tLinch\tWY\tJohnson County\tH1\n82639\t56019\tKaycee\tWY\tJohnson County\tH1\n82009\t56021\tCheyenne\tWY\tLaramie County\tH1\n82059\t56021\tGranite canon\tWY\tLaramie County\tH1\n82001\t56021\tCheyenne\tWY\tLaramie County\tH1\n82003\t56021\tCheyenne\tWY\tLaramie County\tH1\n82050\t56021\tAlbin\tWY\tLaramie County\tH1\n82061\t56021\tHorse creek\tWY\tLaramie County\tH1\n82060\t56021\tHillsdale\tWY\tLaramie County\tH1\n82007\t56021\tCheyenne\tWY\tLaramie County\tH1\n82005\t56021\tFe warren afb\tWY\tLaramie County\tH1\n82052\t56021\tBuford\tWY\tLaramie County\tH1\n82082\t56021\tPine bluffs\tWY\tLaramie County\tH1\n82010\t56021\tCheyenne\tWY\tLaramie County\tH1\n82002\t56021\tCheyenne\tWY\tLaramie County\tH1\n82053\t56021\tBurns\tWY\tLaramie County\tH1\n82054\t56021\tCarpenter\tWY\tLaramie County\tH1\n82081\t56021\tMeriden\tWY\tLaramie County\tH1\n83127\t56023\tThayne\tWY\tLincoln County\tH1\n83110\t56023\tAfton\tWY\tLincoln County\tH1\n83120\t56023\tFreedom\tWY\tLincoln County\tH1\n83118\t56023\tEtna\tWY\tLincoln County\tH1\n83101\t56023\tKemmerer\tWY\tLincoln County\tH1\n83114\t56023\tCokeville\tWY\tLincoln County\tH1\n83126\t56023\tSmoot\tWY\tLincoln County\tH1\n83123\t56023\tLa barge\tWY\tLincoln County\tH1\n83128\t56023\tAlpine\tWY\tLincoln County\tH1\n83122\t56023\tGrover\tWY\tLincoln County\tH1\n83116\t56023\tDiamondville\tWY\tLincoln County\tH1\n83124\t56023\tOpal\tWY\tLincoln County\tH1\n83111\t56023\tAuburn\tWY\tLincoln County\tH1\n83112\t56023\tBedford\tWY\tLincoln County\tH1\n83119\t56023\tFairview\tWY\tLincoln County\tH1\n82605\t56025\tCasper\tWY\tNatrona County\tH1\n82644\t56025\tMills\tWY\tNatrona County\tH1\n82635\t56025\tEdgerton\tWY\tNatrona County\tH1\n82648\t56025\tPowder river\tWY\tNatrona County\tH1\n82636\t56025\tEvansville\tWY\tNatrona County\tH1\n82602\t56025\tCasper\tWY\tNatrona County\tH1\n82604\t56025\tCasper\tWY\tNatrona County\tH1\n82609\t56025\tCasper\tWY\tNatrona County\tH1\n82646\t56025\tNatrona\tWY\tNatrona County\tH1\n82630\t56025\tArminto\tWY\tNatrona County\tH1\n82620\t56025\tAlcova\tWY\tNatrona County\tH1\n82643\t56025\tMidwest\tWY\tNatrona County\tH1\n82601\t56025\tCasper\tWY\tNatrona County\tH1\n82639\t56025\tKaycee\tWY\tNatrona County\tH1\n82701\t56027\tNewcastle\tWY\tNiobrara County\tH1\n82227\t56027\tManville\tWY\tNiobrara County\tH1\n82225\t56027\tLusk\tWY\tNiobrara County\tH1\n82222\t56027\tLance creek\tWY\tNiobrara County\tH1\n82242\t56027\tVan tassell\tWY\tNiobrara County\tH1\n82190\t56029\tYellowstone national park\tWY\tPark County\tH1\n82421\t56029\tDeaver\tWY\tPark County\tH1\n82414\t56029\tCody\tWY\tPark County\tH1\n82411\t56029\tBurlington\tWY\tPark County\tH1\n82433\t56029\tMeeteetse\tWY\tPark County\tH1\n82440\t56029\tRalston\tWY\tPark County\tH1\n82450\t56029\tWapiti\tWY\tPark County\tH1\n82435\t56029\tPowell\tWY\tPark County\tH1\n82214\t56031\tGuernsey\tWY\tPlatte County\tH1\n82201\t56031\tWheatland\tWY\tPlatte County\tH1\n82213\t56031\tGlendo\tWY\tPlatte County\tH1\n82215\t56031\tHartville\tWY\tPlatte County\tH1\n82210\t56031\tChugwater\tWY\tPlatte County\tH1\n82832\t56033\tBanner\tWY\tSheridan County\tH1\n82835\t56033\tClearmont\tWY\tSheridan County\tH1\n82838\t56033\tParkman\tWY\tSheridan County\tH1\n82839\t56033\tRanchester\tWY\tSheridan County\tH1\n82831\t56033\tArvada\tWY\tSheridan County\tH1\n82833
